vi "Init Hardware.vi"(8 "error in (no error)":errorcluster, 11 "NI-Scope Lock-in Driver in":refnum<class "NI-Scope Lock-in Driver.lvclass">) -> (0 "error out":errorcluster, 3 "NI-Scope Lock-in Driver out":refnum<class "NI-Scope Lock-in Driver.lvclass">)   [LabVIEW 2016, in "NI-Scope Lock-in Driver.lvclass"]
uses:
  NI-Scope Lock-in Driver.lvclass
  C:/github/NHMFL_Core/Libraries/NI-DAQ/NI-Scope Digitizer/Ni-Scope Digitizer.lvclass
  NI-Scope Digitizer/Ni-Scope Digitizer.lvclass/Ni-Scope Digitizer.ctl
  NI-Scope Lock-in Driver.lvclass/NI-Scope Lock-in Driver.ctl
  NI-Scope Digitizer/Write Fetch Relative To.vi
  Write Sine.vi
  Write Cosine.vi
  NI-Scope Digitizer/Write Triggering.vi
  NI-Scope Digitizer/Read instrument handle.vi
  NI-Scope Digitizer/Write instrument handle.vi
  NI-Scope Digitizer/Ni-Scope Digitizer.lvclass
  <vilib>/Analysis/NI_AALBase.lvlib
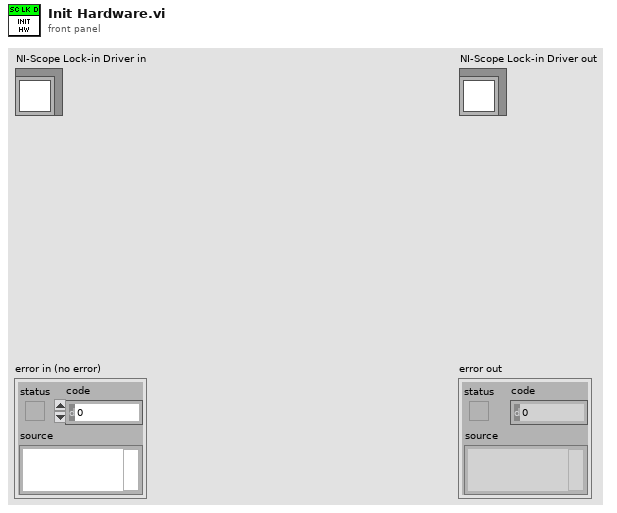
[diagram p1: front panel]
types:
  T1 = typedef "NI-Scope Lock-in Configuration.ctl" = cluster{"Points per sine wave":i32, "Rate":dbl, "Re-name channels":string[], "Active channels":string, "Ranges":dbl[], "Sync on trigger":bool, "R-Q":bool}
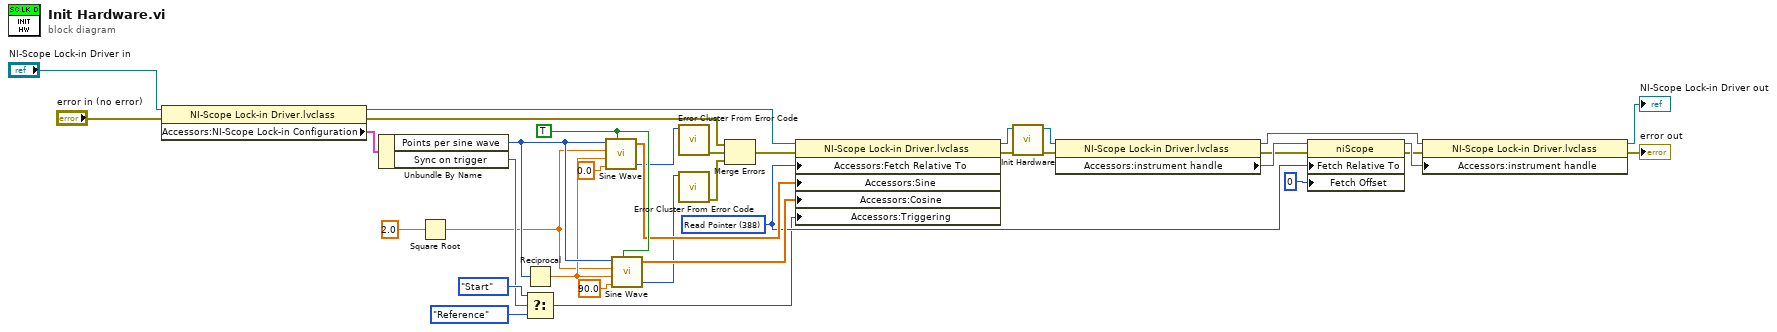
[diagram p0: block diagram]
diagram:
  w29 = TRUE ("reset phase")
  w13 = 388 items=["Start"=482, "Trigger"=483, "Pretrigger"=477, "Now"=481, "Read Pointer"=388] ("Fetch:Fetch Relative To")
  n1 = property class="NI-Scope Lock-in Driver.lvclass"(reference="NI-Scope Lock-in Driver in", error in="error in (no error)") -> (reference out=w31:refnum<class "NI-Scope Lock-in Driver.lvclass">, error out=w33:errorcluster, "Accessors:NI-Scope Lock-in Configuration"=w30:T1)
  n2 = Unbundle By Name(w30) -> ("Points per sine wave"=w26:i32, "Sync on trigger"=w3:bool)
  n3 = Square Root(x=2.0) -> (sqrt(x)=w1:dbl)
  n4 = Reciprocal(x=w26) -> (1/x=w25:dbl)
  n5 = Select(t=enum16{"Reference", "Start"}."Start" ("Triggering"), s=w3, f=enum16{"Reference", "Start"}."Reference" ("Triggering")) -> (s? t:f=w4:enum16{"Reference", "Start"})
  n6 = call <vilib>:"Sine Wave.vi"("samples"=w26, "amplitude"=w1, "frequency"=w25, "phase in"=0.0, "reset phase"=w29) -> ("sine wave"=w23:dbl[], "error"=w21:i32)  [unwired: 1 out]
  n7 = call <vilib>:"Sine Wave.vi"("samples"=w26, "amplitude"=w1, "frequency"=w25, "phase in"=90.0 ("y"), "reset phase"=w29) -> ("sine wave"=w22:dbl[], "error"=w20:i32)  [unwired: 1 out]
  n8 = call <vilib>:"Error Cluster From Error Code.vi"("error code (0)"=w21) -> ("error out"=w18:errorcluster)  [unwired: 8 in]
  n9 = call <vilib>:"Error Cluster From Error Code.vi"("error code (0)"=w20) -> ("error out"=w17:errorcluster)  [unwired: 8 in]
  n10 = Merge Errors(w33, w18, w17) -> (w19:errorcluster)
  n11 = property class="NI-Scope Lock-in Driver.lvclass"(reference=w31, error in=w19, "Accessors:Fetch Relative To"=w13, "Accessors:Sine"=w23, "Accessors:Cosine"=w22, "Accessors:Triggering"=w4) -> (reference out=w34:refnum<class "NI-Scope Lock-in Driver.lvclass">, error out=w35:errorcluster)
  n12 = call-parent "Init Hardware.vi"("error in (no error)"=w35, "Ni-Scope Digitizer in"=w34) -> ("error out"=w15:errorcluster, "Ni-Scope Digitizer out"=w16:refnum<class "NI-Scope Lock-in Driver.lvclass">)  [unwired: 8 in]
  n13 = property class="NI-Scope Lock-in Driver.lvclass"(reference=w16, error in=w15) -> (reference out=w8:refnum<class "NI-Scope Lock-in Driver.lvclass">, error out=w11:errorcluster, "Accessors:instrument handle"=w14:refnum<k15>)
  n14 = property class="niScope"(reference=w14, error in=w11, "Fetch Relative To"=w13, "Fetch Offset"=0 ("Fetch:Fetch Offset")) -> (reference out=w10:refnum<k15>, error out=w9:errorcluster)
  n15 = property class="NI-Scope Lock-in Driver.lvclass"(reference=w8, error in=w9, "Accessors:instrument handle"=w10) -> (reference out=→"NI-Scope Lock-in Driver out":refnum<class "NI-Scope Lock-in Driver.lvclass">, error out=→"error out":errorcluster)
